vi "Check Configuration MD5.vi"(8 "error in (no error)":errorcluster, 11 "Item Ref in":T1 format="%.0x") -> (0 "error out":errorcluster, 3 "Item Ref out":T1 format="%.0x")   [LabVIEW 2017, in "DSF Engine.lvlib"]
uses:
  DSF Engine.lvlib
  <vilib>/NI Veristand/Custom Device API/Custom Device Item Ref.ctl
  Shared/DSF Shared.lvlib
  <vilib>/NI Veristand/Custom Device API/Custom Device API.lvlib
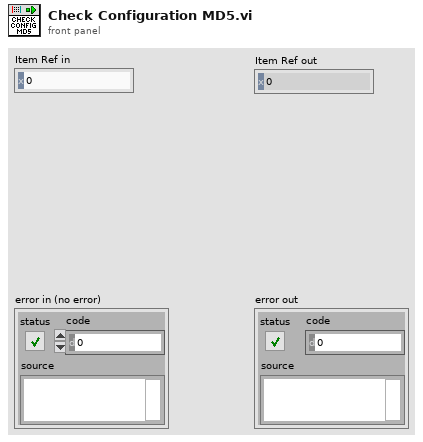
[diagram p1: front panel]
types:
  T1 = typedef "Custom Device API.lvlib/Custom Device Item Ref.ctl" = u64
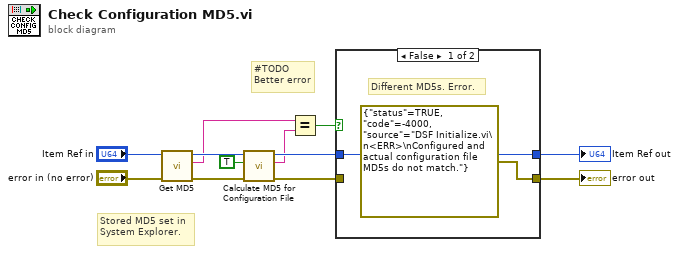
[diagram p0: block diagram]
diagram:
  # "Stored MD5 set in System Explorer."
  # "#TODO\nBetter error"
  n1 = call "Get MD5.vi"("error in (no error)"="error in (no error)", "Item Ref in"="Item Ref in") -> ("error out"=w12:errorcluster, "MD5"=w7:string, "Item Ref out"=w11:T1)  [unwired: 7 in]
  n2 = call "Calculate MD5 for Configuration File.vi"("error in (no error)"=w12, "runtime? (F)"=TRUE, "Item Ref in"=w11) -> ("error out"=w5:errorcluster, "MD5"=w3:string, "Device Ref out"=w4:T1)  [unwired: 6 in]
  n3 = Equal?(x=w7, y=w3) -> (x = y?=w6:bool)
  n4 = case shown="False" w6 {
    tunnel: w5 -> [_ w16]
    tunnel: w4 -> [w14 w15]
    tunnel: [errorcluster {"status"=TRUE, "code"=-4000, "source"="DSF Initialize.vi\n<ERR>\nConfigured and actual configuration file MD5s do not match."} ("error out") w16] -> w2
    tunnel: [w14 w15] -> w1
    frame False {
      # "Different MD5s. Error."
    }
    frame True {
      # "MD5s match. Continue."
    }
  }
  "Item Ref out" <- w1
  "error out" <- w2
